vi "Create ToolStripProgressBar.vi"(8 "error in (no error)":errorcluster caption="错误输入（无错误）", 9 "Width":i32=200, 10 "name":string, 11 "StatusStripClass 输入":refnum<class "StatusStripClass.lvclass"> caption="DNL_LabVIEW Object in") -> (0 "error out":errorcluster caption="错误输出", 2 "ToolStripProgressBar 输出":refnum<class "ToolStripProgressBar.lvclass"> caption="DNL_LabVIEW Object out", 3 "StatusStripClass 输出":refnum<class "StatusStripClass.lvclass"> caption="DNL_LabVIEW Object out")   [LabVIEW 2013, in "StatusStripClass.lvclass"]
uses:
  StatusStripClass.lvclass
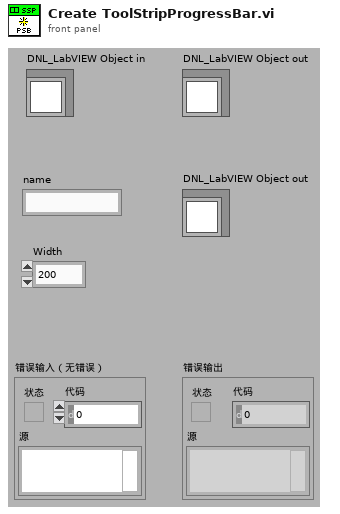
[diagram p1: front panel]
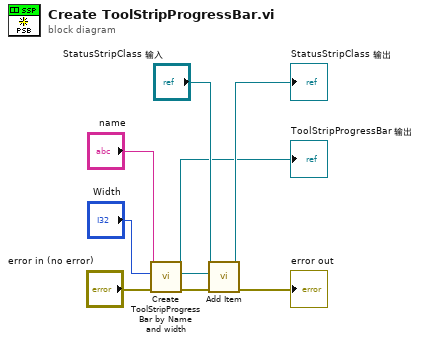
[diagram p0: block diagram]
diagram:
  n1 = call "Create ToolStripProgressBar by Name and width.vi"("error in (no error)"="error in (no error)", "Width"="Width", "name"="name") -> ("error out"=w6:errorcluster, "Item"=w8:refnum<k24>, "ToolStripProgressBar 输出"=→"ToolStripProgressBar 输出":refnum<class "ToolStripProgressBar.lvclass">)  [unwired: 6 in]
  n2 = call "Add Item.vi"("error in (no error)"=w6, "ItemRef"=w8, "StatusStripClass 输入"="StatusStripClass 输入") -> ("error out"=→"error out":errorcluster, "StatusStripClass 输出"=→"StatusStripClass 输出":refnum<class "StatusStripClass.lvclass">)  [unwired: 7 in]
